vi "Cmd Set Parameter Properties (R).vi"(4 "error in (no error)":errorcluster, 5 "parameter properties":T1, 6 "parameter index":variant, 7 "command reference":T4) -> (0 "error out":errorcluster, 3 "command reference out":T4)   [LabVIEW 2013, in "NI_Database_API_64.lvlib"]
doc: "Sets properties on the object as determined by the inputs. This VI works for connections, commands, and parameters. For parameters, a parameter index must be wired to the input below the <B>reference</B>."
uses:
  NI_Database_API_64.lvlib
  Cmd ObjectReference.ctl
  Cmd Parameter Properties.ctl
  Auxilliary.llb/DB Tools DataTypes.ctl
  Auxilliary.llb/DB Tools Parameter Dir.ctl
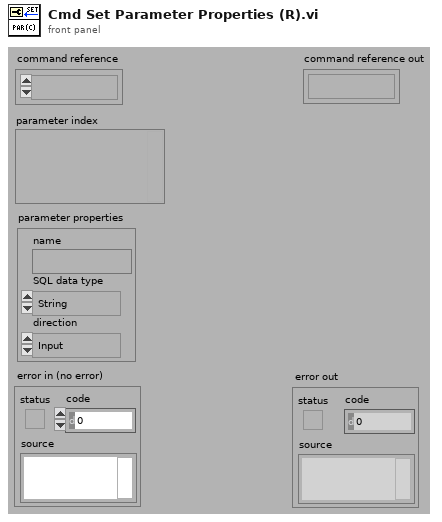
[diagram p1: front panel]
types:
  T1 = typedef "NI_Database_API_64.lvlib/Cmd Parameter Properties.ctl" = cluster{"name":string, "SQL data type":T2, "direction":T3}
  T2 = typedef "NI_Database_API_64.lvlib/DB Tools DataTypes.ctl" = enum16{"String", "Long (I32)", "Single (SGL)", "Double (DBL)", "Date/Time", "Binary"}
  T3 = typedef "NI_Database_API_64.lvlib/DB Tools Parameter Dir.ctl" = enum32{"Input", "Output", "Input/Output", "Return Value"}
  T4 = typedef "NI_Database_API_64.lvlib/Cmd ObjectReference.ctl" = refnum<k1>
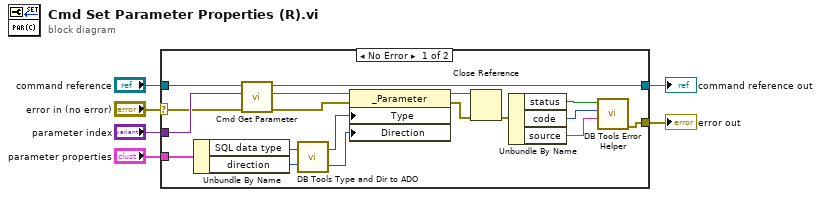
[diagram p0: block diagram]
diagram:
  n1 = case shown="No Error" "error in (no error)" {
    selector: "error in (no error)" -> [w7 w26]
    tunnel: "command reference" -> [w23 w25]
    tunnel: "parameter index" -> [w22 _]
    tunnel: [w21 w25] -> w4
    tunnel: "parameter properties" -> [w18 _]
    tunnel: [w8 w26] -> w2
    frame No Error {
      n2 = Unbundle By Name(w18) -> ("SQL data type"=w17:T2, "direction"=w16:T3)
      n3 = call "Cmd Get Parameter.vi"("error in (no error)"=w7, "parameter index"=w22, "command reference"=w23) -> ("error out"=w19:errorcluster, "ADODB.Parameter"=w20:refnum<k7>, "command reference out"=w21:T4)  [unwired: 2 out]
      n4 = call "DB Tools Type and Dir to ADO.vi"("direction"=w16, "data type"=w17) -> ("ADO direction"=w14:u16, "ADO type"=w15:u16)
      n5 = property class="_Parameter"(reference=w20, error in=w19, "Type"=w15, "Direction"=w14) -> (reference out=w24:refnum<k7>, error out=w13:errorcluster)
      n6 = Close Reference(reference=w24, error in (no error)=w13) -> (error out=w9:errorcluster)
      n7 = Unbundle By Name(w9) -> ("status"=w11:bool, "code"=w10:i32, "source"=w12:string)
      n8 = call "DB Tools Error Helper.vi"("source"=w12, "code"=w10, "status"=w11) -> ("error out"=w8:errorcluster)  [unwired: 1 in, 7 out]
    }
    frame Error {
    }
  }
  "command reference out" <- w4
  "error out" <- w2
